vi "Close Device.vi"(8 "error in (no error)":errorcluster, 11 "Toggle 8 (niDig) in":refnum<class "Toggle 8 (niDig).lvclass">) -> (0 "error out":errorcluster, 3 "Toggle 8 (niDig) out":refnum<class "Toggle 8 (niDig).lvclass">)   [LabVIEW 2020, in "Toggle 8 (niDig).lvclass"]
uses:
  Toggle 8 (niDig).lvclass
  niDigital.lvclass
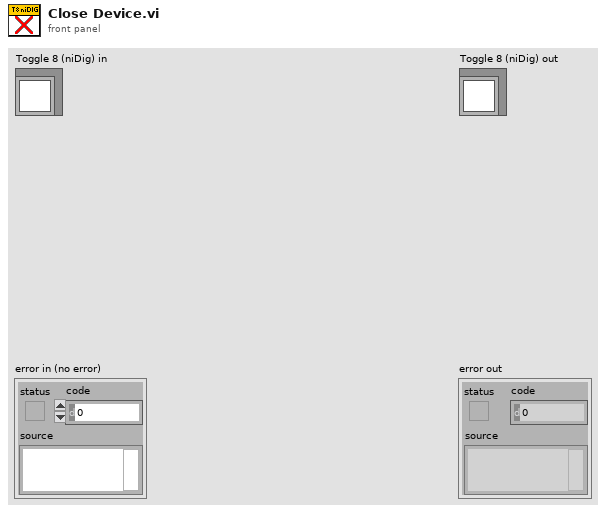
[diagram p1: front panel]
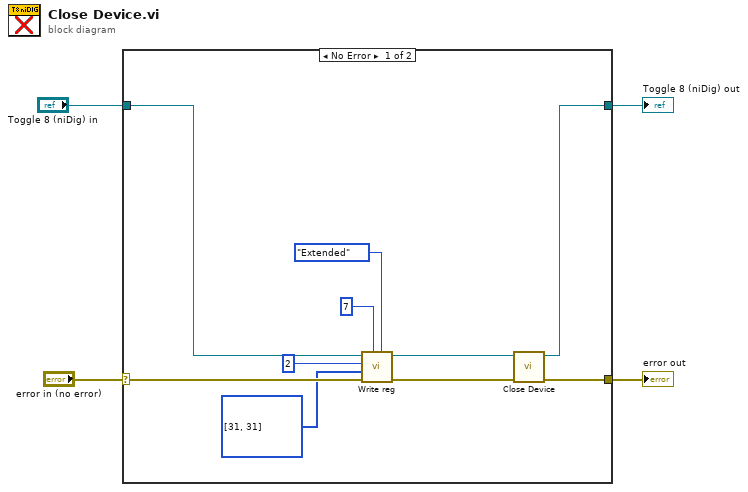
[diagram p0: block diagram]
diagram:
  n1 = case shown="No Error" "error in (no error)" {
    selector: "error in (no error)" -> [w12 w16]
    tunnel: [w14 w16] -> w4
    tunnel: [w13 w15] -> w3
    tunnel: "Toggle 8 (niDig) in" -> [w7 w15]
    frame No Error {
      n2 = call-dynamic "Write reg.vi"("Write type"=enum16{"Normal", "Extended", "Extended Cycle"}."Extended", "Write USID"=u8 7, "error in (no error)"=w12, "Write Data"=u32[] [31, 31], "Write Address"=u32 2, "niDigital in"=w7) -> ("error out"=w11:errorcluster, "niDigital out"=w10:refnum<class "Toggle 8 (niDig).lvclass">)  [unwired: 4 in]
      n3 = call-parent "Close Device.vi"("error in (no error)"=w11, "niDigital in"=w10) -> ("error out"=w14:errorcluster, "niDigital out"=w13:refnum<class "Toggle 8 (niDig).lvclass">)  [unwired: 8 in]
    }
    frame Error {
    }
  }
  "error out" <- w4
  "Toggle 8 (niDig) out" <- w3
